vi "MFLI_set_freq-and-get--V1.vi"(4 "Oscillator (0)":u16, 6 "delay-circle(msec)":i64, 8 "Error In":errorcluster, 9 "timeconstant (s)":dbl=0.006, 10 "Freq in (Hz)":dbl=40000.0 format="%#_13g", 11 "Handle In":T1 {"Handle" format="0x%08x"; "Conn" format="0x%08x"}) -> (0 "Error Out":errorcluster, 1 "z out (V)":cdb, 2 "Freq out (Hz)":dbl=40000.0 format="%#_13g", 3 "Handle Out":T1 {"Handle" format="0x%08x"; "Conn" format="0x%08x"})   [LabVIEW 2018]
uses:
  Applications/National Instruments/LabVIEW 2019 64-bit/instr.lib/Zurich Instruments LabOne/Zurich Instruments LabOne.lvlib
  Applications/National Instruments/LabVIEW 2019 64-bit/instr.lib/Zurich Instruments LabOne/Public/ziTypeHandle.ctl
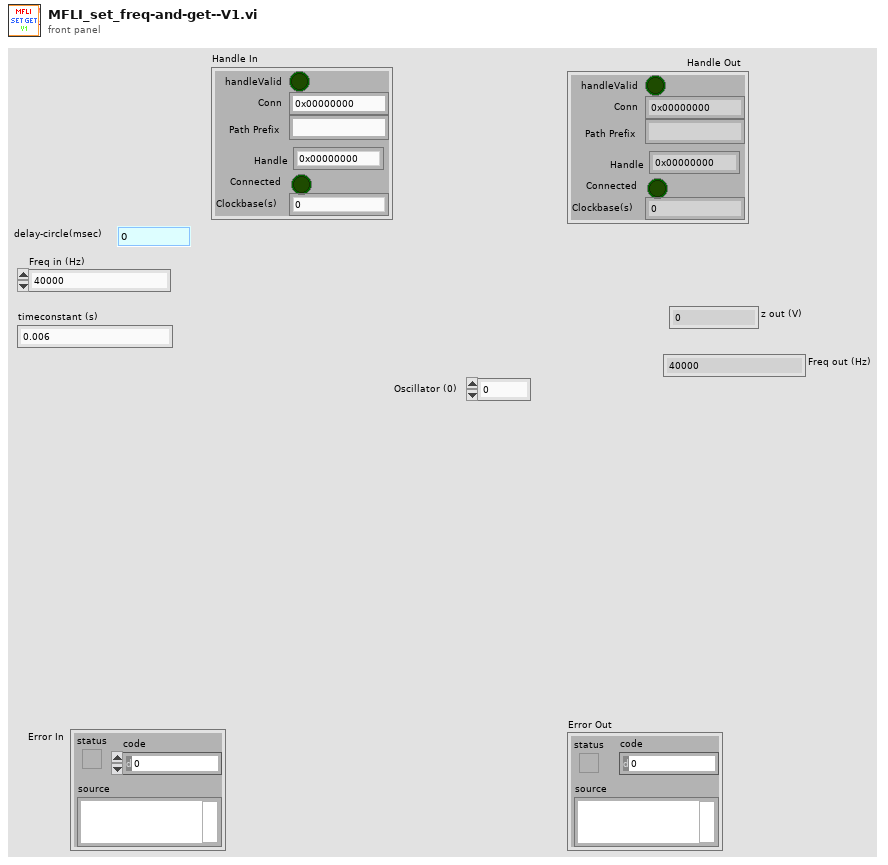
[diagram p1: front panel]
types:
  T1 = typedef "Zurich Instruments LabOne.lvlib/ziTypeHandle.ctl" = cluster{"handleValid":bool, "Conn":u64, "Path Prefix":string, "Handle":u64, "Connected":bool, "Clockbase(s)":dbl}
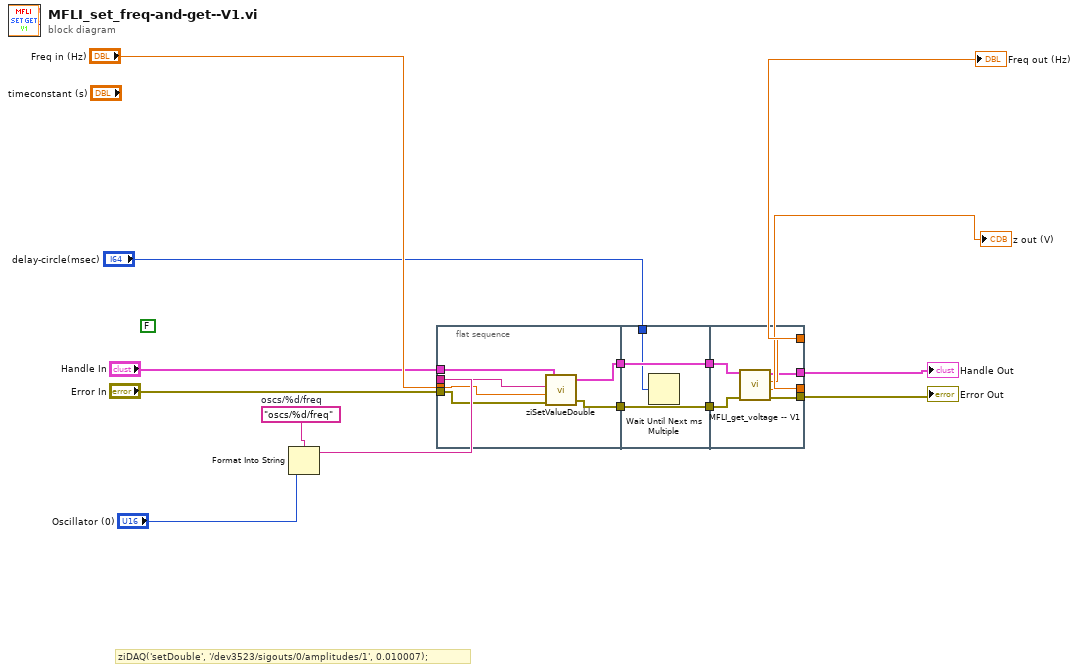
[diagram p0: block diagram]
diagram:
  (unwired) FALSE
  w15 = "oscs/%d/freq"  # oscs/%d/freq
  # "ziDAQ('setDouble', '/dev3523/sigouts/0/amplitudes/1', 0.010007);"
  n1 = Format Into String(format string=w15, "Oscillator (0)") -> (resulting string=w14:string)  [unwired: 2 in, 1 out]
  n2 = flat-sequence {
    tunnel: w14 -> [w21]
    tunnel: "Freq in (Hz)" -> [w20]
    tunnel: "Handle In" -> [w19]
    tunnel: "Error In" -> [w18]
    tunnel: [w17] -> w5
    tunnel: [w16] -> w3
    tunnel: w5 -> [w24]
    tunnel: [w24] -> w4
    tunnel: w3 -> [w23]
    tunnel: [w23] -> w2
    tunnel: "delay-circle(msec)" -> [w22]
    tunnel: [w27] -> w6
    tunnel: [w26] -> w7
    tunnel: [w25] -> w8
    tunnel: [w28] -> w9
    tunnel: w4 -> [w30]
    tunnel: w2 -> [w29]
    frame #0 {
      n3 = call "ziSetValueDouble.vi"("Error In"=w18, "Value"=w20, "Path"=w21, "Handle In"=w19) -> ("Error Out"=w17:errorcluster, "Handle Out"=w16:T1)  [unwired: 1 in]
    }
    frame #1 {
      n4 = Wait Until Next ms Multiple(millisecond multiple=w22) -> ()  [unwired: 1 out]
    }
    frame #2 {
      n5 = call "MFLI_get_voltage -- V1.vi"("Error In"=w30, "Handle In"=w29) -> ("Error Out"=w28:errorcluster, "z out (V)"=w27:cdb, "Freq out (Hz)"=w26:dbl, "Handle Out"=w25:T1)  [unwired: 6 in]
    }
  }
  "Handle Out" <- w8
  "Error Out" <- w9
  "z out (V)" <- w6
  "Freq out (Hz)" <- w7
